vi "Display Settings.vi"(10 "ref":refnum<vi>) -> ()   [LabVIEW 2009, in "POLARIS IMAQ Display.xctl"]
uses:
  POLARIS IMAQ Display.xctl
  DisplaySettings.ctl
panel:
  in  "Stop":bool
  in  "Display settings":T1={"Min. Thresh."=0.0, "X"=0.0, "Y"=0.0, "ShowLineout"=FALSE, "ScaleParts"=10, "ShowLegende"=FALSE, "Target Cross"=FALSE, "Centroid Cross"=FALSE, "Target color"=16777226, "Centroid color"=16711680, "calibr. mm/px"=0.0}
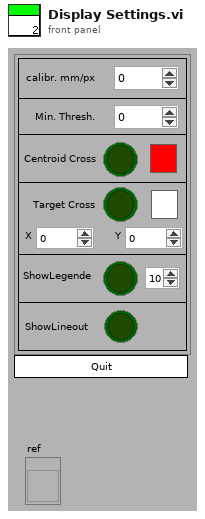
[diagram p1: front panel]
types:
  T1 = typedef "POLARIS IMAQ Display.xctl/DisplaySettings.ctl" = cluster{"Min. Thresh.":sgl, "X":dbl, "Y":dbl, "ShowLineout":bool, "ScaleParts":i32, "ShowLegende":bool, "Target Cross":bool, "Centroid Cross":bool, "Target color":u32, "Centroid color":u32, "calibr. mm/px":sgl}
  T2 = cluster{"Min. Thresh.":sgl, "X":dbl, "Y":dbl, "ShowLineout":bool, "ScaleParts":i32, "ShowLegende":bool, "Target Cross":bool, "Centroid Cross":bool, "Target color":u32, "Centroid color":u32, "calibr. mm/px":sgl}
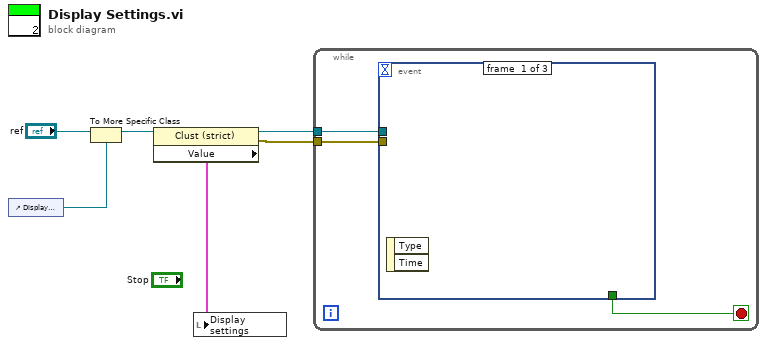
[diagram p0: block diagram]
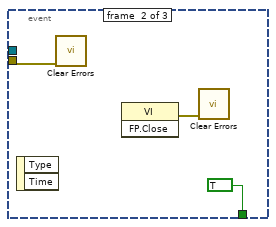
[diagram p2: hidden frame]
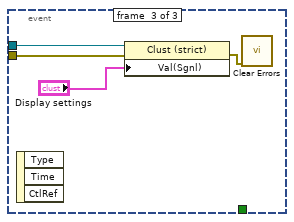
[diagram p3: hidden frame]
diagram:
  n1 = control-ref of="Display settings"() -> (w5:refnum<vi>)
  n2 = To More Specific Class(target class=w5, reference="ref") -> (specific class reference=w4:refnum<vi>)  [unwired: 1 in, 1 out]
  n3 = property class="Clust (strict)"(reference=w4) -> (reference out=w3:refnum<vi>, error out=w1:errorcluster, "Value"=w2:T2)  [unwired: 1 in]
  n4 = local write "Display settings"(w2) -> ()
  n5 = while {
    tunnel: w3 -> [w8]
    tunnel: w1 -> [w7]
    stop <- w9 stop-if-true
    n6 = event shown="[1] \"Stop\": Value Change;  Application Instance Close" {
      selector: _ -> [_ _ _]
      dyn-events: _ -> [_ _ _]
      timeout: _ -> [_ _ _]
      tunnel: [_ TRUE _] -> w9
      tunnel: w8 -> [_ _ w15]
      tunnel: w7 -> [_ w11 w14]
      event #0 {
        n7 = event-data() -> ()  [unwired: 1 in, 2 out]
      }
      event #1 {
        n8 = event-data() -> ()  [unwired: 1 in, 2 out]
        n9 = call <vilib>:"Clear Errors.vi"("error in (no error)"=w11) -> ()  [unwired: 6 in, 1 out]
        n10 = invoke class="VI" method="FP.Close"() -> (error out=w10:errorcluster)  [unwired: 3 in, 2 out]
        n11 = call <vilib>:"Clear Errors.vi"("error in (no error)"=w10) -> ()  [unwired: 6 in, 1 out]
      }
      event #2 {
        n12 = event-data() -> ()  [unwired: 1 in, 3 out]
        n13 = property class="Clust (strict)"(reference=w15, error in=w14, "Val(Sgnl)"="Display settings") -> (error out=w13:errorcluster)  [unwired: 1 out]
        n14 = call <vilib>:"Clear Errors.vi"("error in (no error)"=w13) -> ()  [unwired: 6 in, 1 out]
      }
    }
  }
